vi "LOAD CELL MAIN CODE.vi"() -> ()   [LabVIEW 2025]
panel:
  in  "Case Constant\n(See Context Help) 3":bool=TRUE
  in  "Case Constant\n(See Context Help) 2":bool=TRUE
  in  "Case Constant\n(See Context Help)":bool
  in  "Acq Delay :":u32=20
  in  "FILE PATH":path
  in  "MODEL :":string
  out "LOAD CELL STATUS":bool
  in  "Start":bool=TRUE
  in  "stop":bool
  in  "Tab Control":T1(tab)
  in  "FILE NAME":string
  in  "Load cell parameter set":bool
  in  "SN":string="0"
  in  "ft_udp_handle":string="0"
  in  "PORT NO":string="8080"
  in  "IP ADDRESS":string="192.168.1.100"
  out "Fx":dbl(graph)
  out "Fy":dbl(graph)
  out "Fz":dbl(graph)
  out "Mx":dbl(graph)
  out "Mz":dbl(graph)
  out "My":dbl(graph)
  out "error out":errorcluster
  in  "error in (no error)":errorcluster
  out "model":string
  # "LOAD CELL DATA MONITOR"
types:
  T1 = enum32{"Instrument Details", "Fx", "Fy", "Fz", "Mx", "My", "Mz"}
  T2 = enum16{"INIT", "MAIN", "SET", "READ DATA", "CLOSE"}
  T3 = cluster{"load cell fgv ref":cluster{"Sensor IP":string, "Port":i32, "SN":i32, "model":string, "deleteHandle-result":i32, "initial-return":i32, "filter-return":i32, "zero-return":i32, "get-range-return":i32, "get-data-return":i32, "ft_udp_handle":i32, "ft_data":dbl[], "ft_range":dbl[], "running_flag":bool, "Create Handle":bool, "delete Handle":bool, "AE":bool, "uninitial-return":i32}, "main screen ref":cluster{"Fz":dbl, "Fy":dbl, "Fx":dbl, "Start":bool, "stop":bool, "IP ADDRESS":string, "PORT NO":string, "ft_udp_handle":string, "SN":string, "LOAD CELL STATUS":bool, "Load cell parameter set":bool, "FILE PATH":path, "MODEL :":string, "FILE NAME":string, "Tab Control":enum32{"Instrument Details", "Fx", "Fy", "Fz", "Mx", "My", "Mz"}, "Mz":dbl, "My":dbl, "Mx":dbl}}
  T4 = enum16{"INIT", "SETLOWPASSFILTER", "SETZERO", "GETSENSORINFO", "GETRANGE", "ZEROALL", "READDATA", "UNINITIAL", "DELETEHANDLE"}
  T5 = cluster{"Sensor IP":string, "Port":i32, "SN":i32, "model":string, "deleteHandle-result":i32, "initial-return":i32, "filter-return":i32, "zero-return":i32, "get-range-return":i32, "get-data-return":i32, "ft_udp_handle":i32, "ft_data":dbl[], "ft_range":dbl[], "running_flag":bool, "Create Handle":bool, "delete Handle":bool, "AE":bool, "uninitial-return":i32}
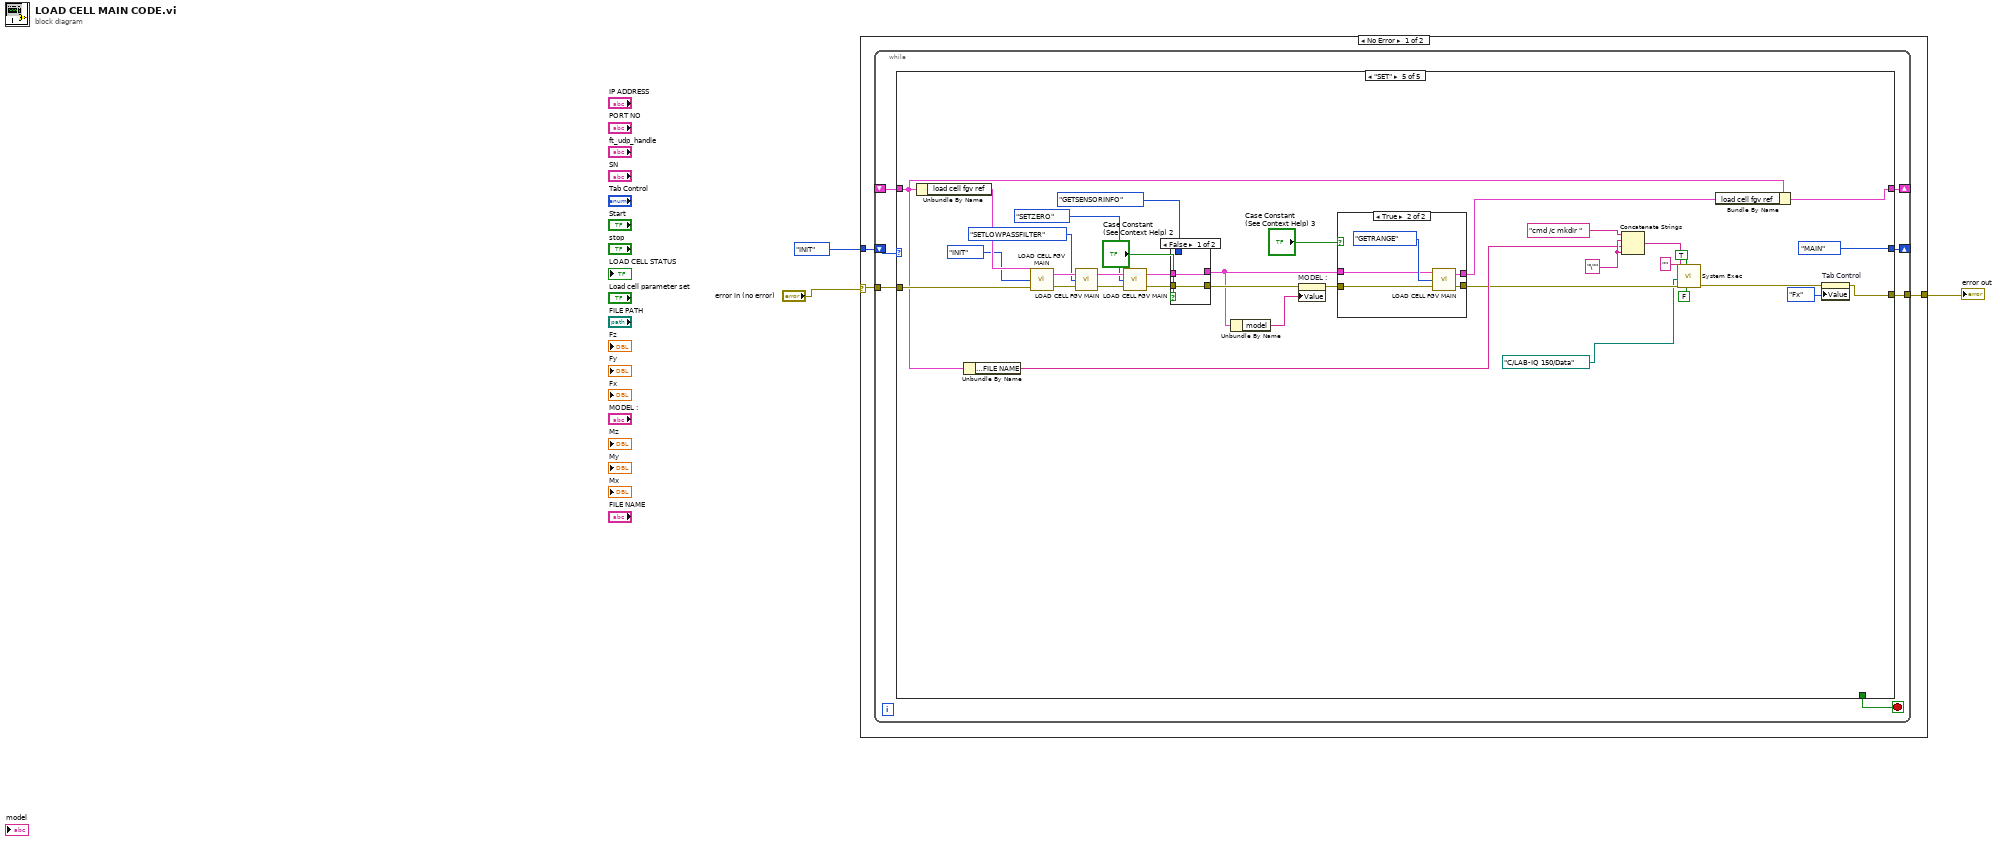
[diagram p0: block diagram]
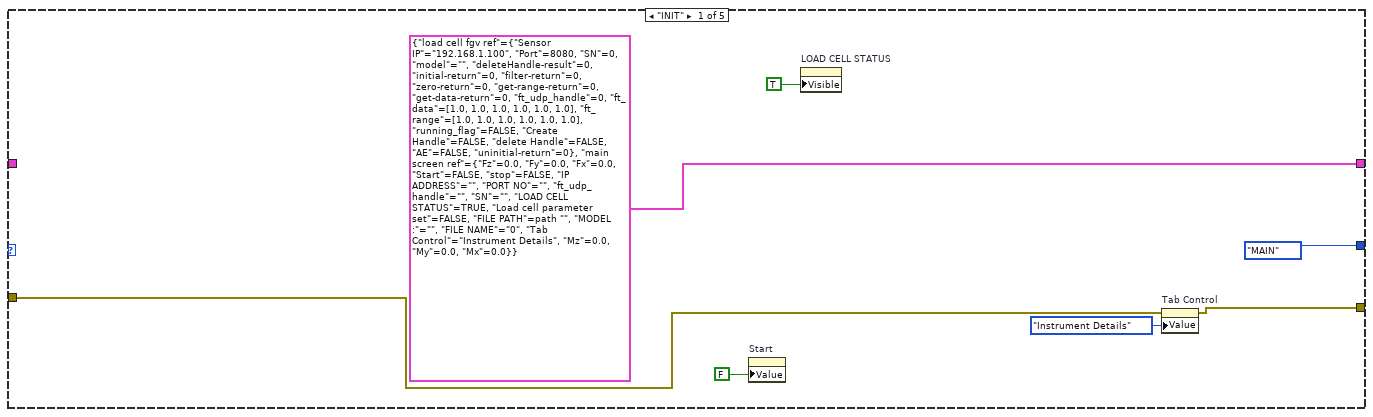
[diagram p2: hidden frame]
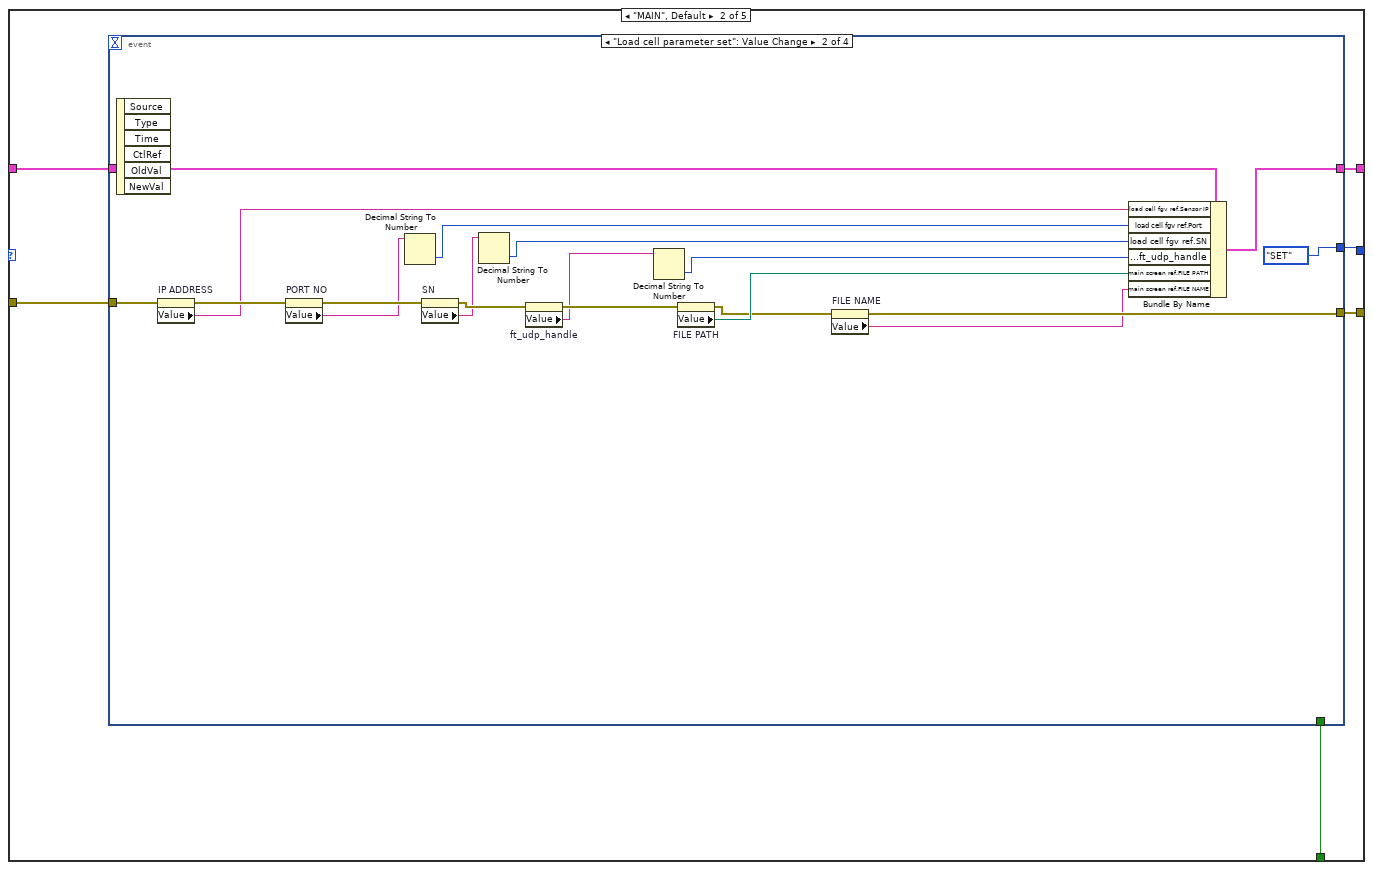
[diagram p3: hidden frame]
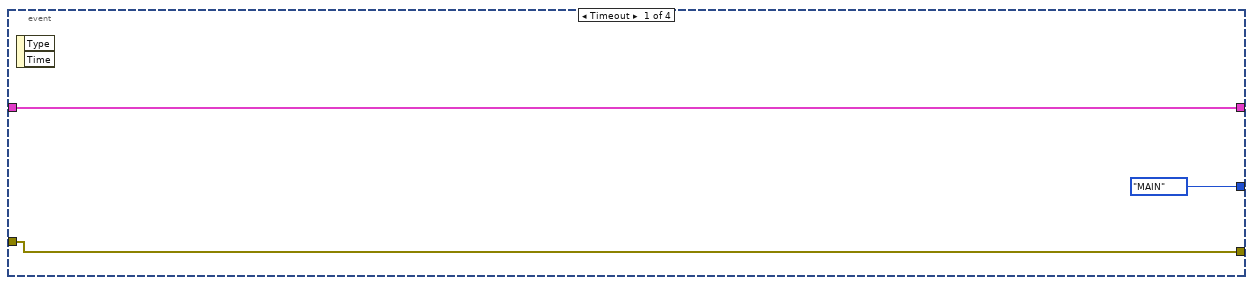
[diagram p4: hidden frame]
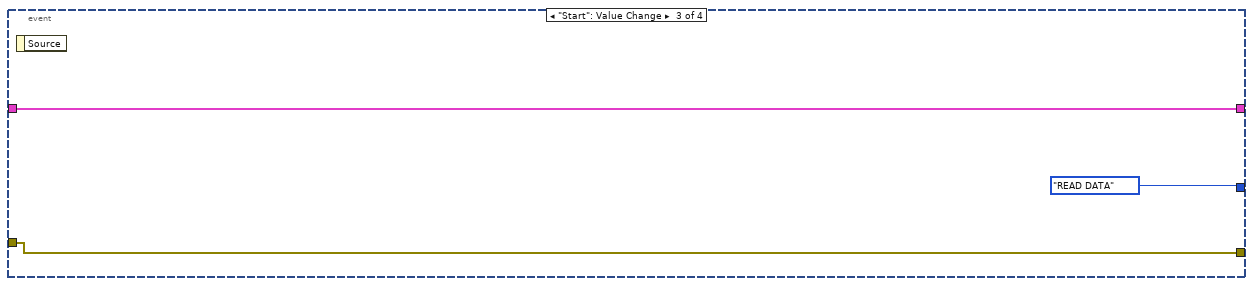
[diagram p5: hidden frame]
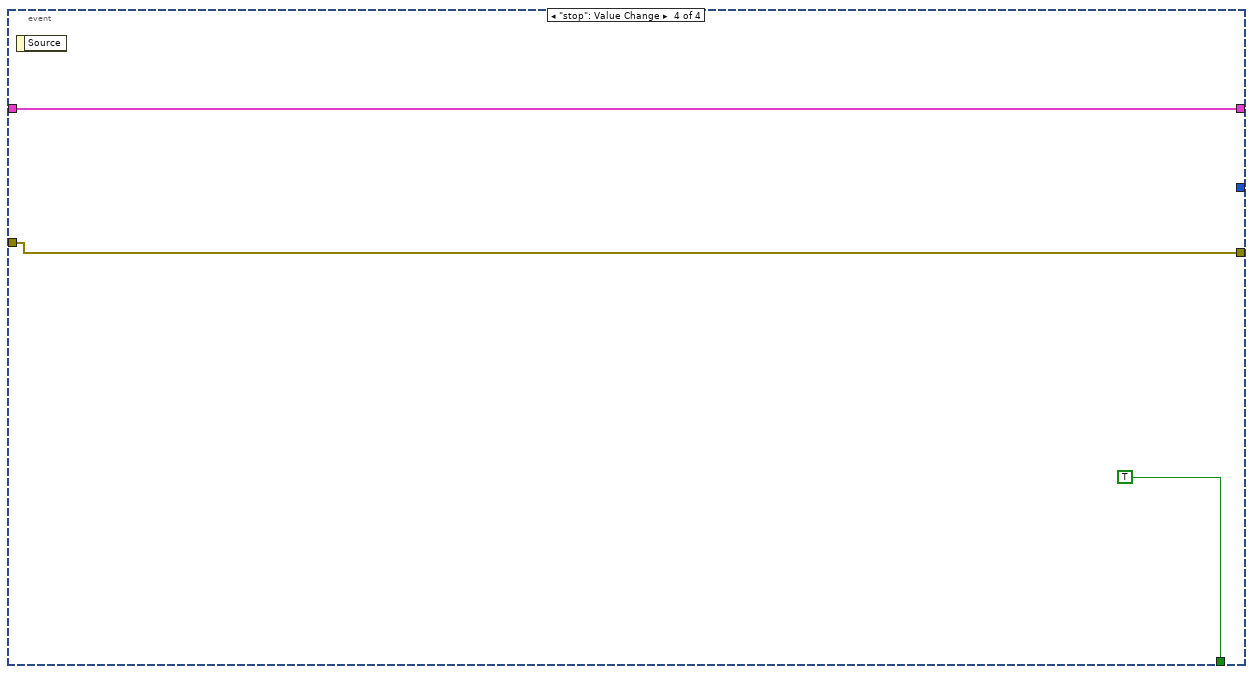
[diagram p6: hidden frame]
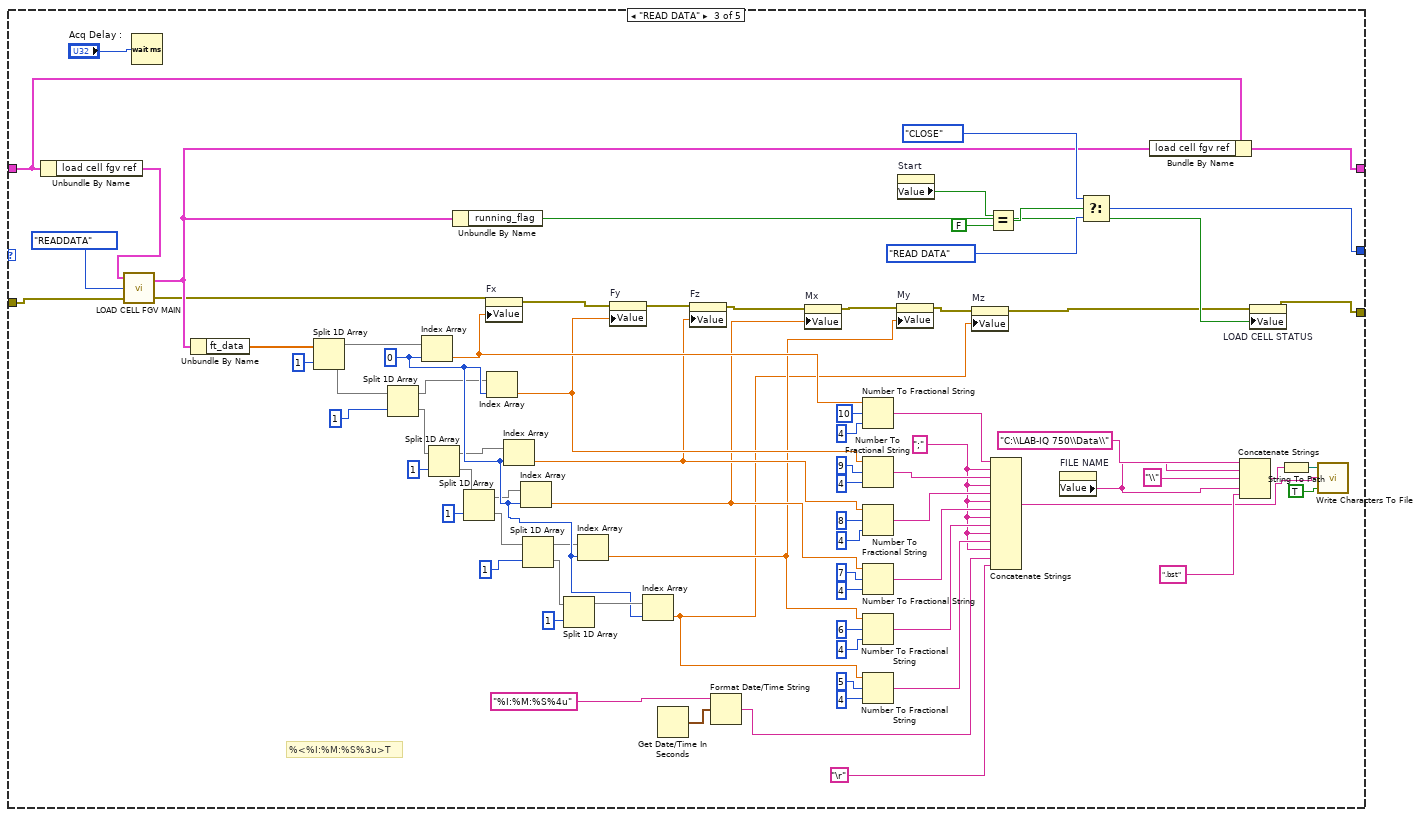
[diagram p7: hidden frame]
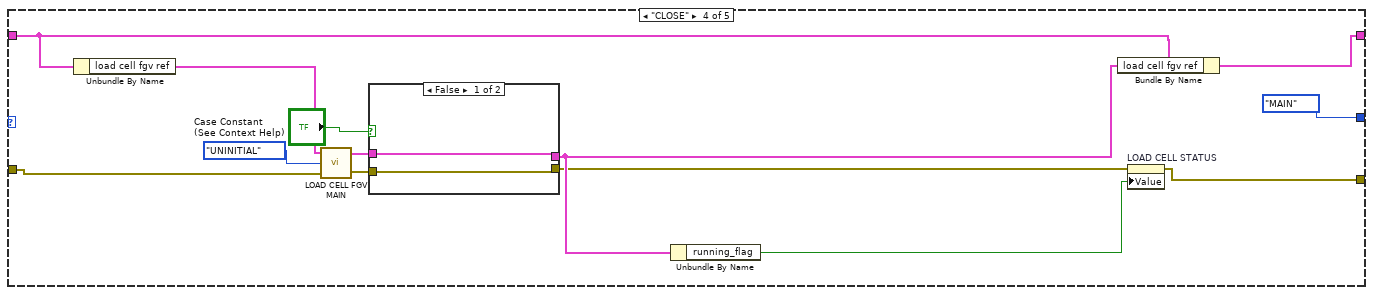
[diagram p8: hidden frame]
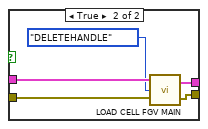
[diagram p9: hidden frame]
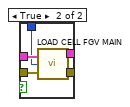
[diagram p11: hidden frame]
diagram:
  n1 = case shown="No Error" "error in (no error)" {
    selector: "error in (no error)" -> [w5 w201]
    tunnel: [w4 w201] -> w2
    tunnel: T2."INIT" -> [w6 _]
    frame No Error {
      n2 = while {
        shift-right: [w9] -> _
        shift-left: w6 -> [w13]
        tunnel: w5 -> [w12]
        shift-right: [w10] -> _
        shift-left: _ -> [w11]
        tunnel: [w8] -> w4
        stop <- w7 stop-if-true
        n3 = case shown="\"SET\"" w13 {
          tunnel: w12 -> [w17 w26 w132 w144 w186]
          tunnel: w11 -> [_ w23 w122 w142 w165]
          tunnel: [T3 {"load cell fgv ref"={"Sensor IP"="192.168.1.100", "Port"=8080, "SN"=0, "model"="", "deleteHandle-result"=0, "initial-return"=0, "filter-return"=0, "zero-return"=0, "get-range-return"=0, "get-data-return"=0, "ft_udp_handle"=0, "ft_data"=[1.0, 1.0, 1.0, 1.0, 1.0, 1.0], "ft_range"=[1.0, 1.0, 1.0, 1.0, 1.0, 1.0], "running_flag"=FALSE, "Create Handle"=FALSE, "delete Handle"=FALSE, "AE"=FALSE, "uninitial-return"=0}, "main screen ref"={"Fz"=0.0, "Fy"=0.0, "Fx"=0.0, "Start"=FALSE, "stop"=FALSE, "IP ADDRESS"="", "PORT NO"="", "ft_udp_handle"="", "SN"="", "LOAD CELL STATUS"=TRUE, "Load cell parameter set"=FALSE, "FILE PATH"=path "", "MODEL :"="", "FILE NAME"="0", "Tab Control"=enum."Instrument Details", "Mz"=0.0, "My"=0.0, "Mx"=0.0}} w24 w123 w141 w178] -> w10
          tunnel: [T2."MAIN" w25 w124 T2."MAIN" T2."MAIN"] -> w9
          tunnel: [w18 w22 w113 w134 w166] -> w8
          tunnel: [_ w21 _ _ _] -> w7
          frame "INIT" {
            n4 = property on="Start" class="Bool (strict)"("Value"=FALSE ("Start")) -> ()  [unwired: 2 in, 2 out]
            n5 = property on="LOAD CELL STATUS" class="Bool (strict)"("Visible"=TRUE) -> ()  [unwired: 2 in, 2 out]
            n6 = property on="Tab Control" class="TabCtl (strict)"(error in=w17, "Value"=enum32{"Instrument Details", "Fx", "Fy", "Fz"}."Instrument Details" ("Tab Control")) -> (error out=w18:errorcluster)  [unwired: 1 in, 1 out]
          }
          frame "MAIN", Default {
            n7 = event shown="[1] \"Load cell parameter set\": Value Change" {
              selector: _ -> [_ _ _ _]
              dyn-events: _ -> [_ _ _ _]
              timeout: _ -> [_ _ _ _]
              tunnel: w26 -> [w28 w48 w51 w54]
              tunnel: [T2."MAIN" T2."SET" T2."READ DATA" _] -> w25
              tunnel: [w27 w42 w49 w52] -> w24
              tunnel: w23 -> [w27 w43 w49 w52]
              tunnel: [w28 w37 w51 w54] -> w22
              tunnel: [_ _ _ TRUE] -> w21
              event Timeout {
                n8 = event-data() -> ()  [unwired: 1 in, 2 out]
              }
              event "Load cell parameter set": Value Change {
                n9 = event-data() -> ()  [unwired: 1 in, 6 out]
                n10 = property on="IP ADDRESS" class="Str"(error in=w48) -> (error out=w47:errorcluster, "Value"=w40:string)  [unwired: 1 in, 1 out]
                n11 = property on="PORT NO" class="Str"(error in=w47) -> (error out=w46:errorcluster, "Value"=w35:string)  [unwired: 1 in, 1 out]
                n12 = Decimal String To Number(string=w35) -> (number=w33:i32)  [unwired: 2 in, 1 out]
                n13 = property on="SN" class="Str"(error in=w46) -> (error out=w45:errorcluster, "Value"=w34:string)  [unwired: 1 in, 1 out]
                n14 = Decimal String To Number(string=w34) -> (number=w32:i32)  [unwired: 2 in, 1 out]
                n15 = property on="ft_udp_handle" class="Str"(error in=w45) -> (error out=w44:errorcluster, "Value"=w31:string)  [unwired: 1 in, 1 out]
                n16 = Decimal String To Number(string=w31) -> (number=w30:i32)  [unwired: 2 in, 1 out]
                n17 = property on="FILE PATH" class="Path"(error in=w44) -> (error out=w38:errorcluster, "Value"=w41:path)  [unwired: 1 in, 1 out]
                n18 = property on="FILE NAME" class="Str"(error in=w38) -> (error out=w37:errorcluster, "Value"=w36:string)  [unwired: 1 in, 1 out]
                n19 = Bundle By Name(cluster=w43, "load cell fgv ref.Sensor IP"=w40, "load cell fgv ref.Port"=w33, "load cell fgv ref.SN"=w32, "load cell fgv ref.ft_udp_handle"=w30, "main screen ref.FILE PATH"=w41, "main screen ref.FILE NAME"=w36) -> (w42:T3)
              }
              event "Start": Value Change {
                n20 = event-data() -> ()  [unwired: 1 in, 1 out]
              }
              event "stop": Value Change {
                n21 = event-data() -> ()  [unwired: 1 in, 1 out]
              }
            }
          }
          frame "READ DATA" {
            w59 = ";" ("F-format string")
            w71 = 0 ("index")
            # "%<%I:%M:%S%3u>T"
            n22 = Unbundle By Name(w122) -> ("load cell fgv ref"=w130:T5)
            n23 = call "LOAD CELL FGV MAIN.vi"("error in (no error)"=w132, "Enum"=T4."READDATA", "Cluster IN 2"=w130) -> ("error IO"=w110:errorcluster, "Cluster IN"=w114:T5)
            n24 = Wait (ms)(milliseconds to wait="Acq Delay :") -> ()  [unwired: 1 out]
            n25 = Unbundle By Name(w114) -> ("ft_data"=w117:dbl[])
            n26 = Split 1D Array(array=w117, index=1) -> (first subarray=w116:dbl[], second subarray=w121:dbl[])
            n27 = Split 1D Array(array=w121, index=1) -> (first subarray=w63:dbl[], second subarray=w115:dbl[])
            n28 = Index Array(array=w116, index=w71) -> (element=w89:dbl)
            n29 = Split 1D Array(array=w115, index=1) -> (first subarray=w62:dbl[], second subarray=w90:dbl[])
            n30 = Unbundle By Name(w114) -> ("running_flag"=w112:bool)
            n31 = Split 1D Array(array=w90, index=1) -> (first subarray=w61:dbl[], second subarray=w74:dbl[])
            n32 = property on="Fx" class="WFChart (strict)"(error in=w110, "Value"=w89) -> (error out=w109:errorcluster)  [unwired: 1 in, 1 out]
            n33 = Index Array(array=w63, index=w71) -> (element=w80:dbl)
            n34 = Index Array(array=w62, index=w71) -> (element=w79:dbl)
            n35 = Index Array(array=w61, index=w71) -> (element=w70:dbl)
            n36 = Split 1D Array(array=w74, index=1) -> (first subarray=w60:dbl[], second subarray=w73:dbl[])
            n37 = Split 1D Array(array=w73, index=1) -> (first subarray=w72:dbl[])  [unwired: 1 out]
            n38 = Index Array(array=w60, index=w71) -> (element=w69:dbl)
            n39 = property on="Fy" class="WFChart (strict)"(error in=w109, "Value"=w80) -> (error out=w108:errorcluster)  [unwired: 1 in, 1 out]
            n40 = Index Array(array=w72, index=w71) -> (element=w68:dbl)
            n41 = Get Date/Time In Seconds() -> (seconds since 1Jan1904=w57:timestamp)
            n42 = property on="Fz" class="WFChart (strict)"(error in=w108, "Value"=w79) -> (error out=w78:errorcluster)  [unwired: 1 in, 1 out]
            n43 = Format Date/Time String(time format string (%c)="%I:%M:%S%4u", seconds (now)=w57) -> (date/time string=w55:string)  [unwired: 1 in]
            n44 = property on="Mx" class="WFChart (strict)"(error in=w78, "Value"=w70) -> (error out=w77:errorcluster)  [unwired: 1 in, 1 out]
            n45 = Number To Fractional String(number=w89, width (-)=i16 10 ("precision (6)"), precision (6)=i16 4) -> (F-format string=w98:string)  [unwired: 1 in]
            n46 = Number To Fractional String(number=w80, width (-)=i16 9 ("precision (6)"), precision (6)=i16 4) -> (F-format string=w99:string)  [unwired: 1 in]
            n47 = Number To Fractional String(number=w79, width (-)=i16 8 ("precision (6)"), precision (6)=i16 4) -> (F-format string=w67:string)  [unwired: 1 in]
            n48 = Number To Fractional String(number=w70, width (-)=i16 7 ("precision (6)"), precision (6)=i16 4) -> (F-format string=w66:string)  [unwired: 1 in]
            n49 = Number To Fractional String(number=w69, width (-)=i16 6 ("precision (6)"), precision (6)=i16 4) -> (F-format string=w65:string)  [unwired: 1 in]
            n50 = Number To Fractional String(number=w68, width (-)=i16 5 ("precision (6)"), precision (6)=i16 4) -> (F-format string=w64:string)  [unwired: 1 in]
            n51 = property on="My" class="WFChart (strict)"(error in=w77, "Value"=w69) -> (error out=w76:errorcluster)  [unwired: 1 in, 1 out]
            n52 = property on="Start" class="Bool (strict)"() -> ("Value"=w129:bool)  [unwired: 2 in, 2 out]
            n53 = property on="Mz" class="WFChart (strict)"(error in=w76, "Value"=w68) -> (error out=w75:errorcluster)  [unwired: 1 in, 1 out]
            n54 = Equal?(x=w129, y=FALSE) -> (x = y?=w127:bool)
            n55 = Concatenate Strings(w98, w59, w99, w59, w67, w59, w66, w59, w65, w59, w64, w59, w55, "\r") -> (w94:string)
            n56 = property on="FILE NAME" class="Str"() -> ("Value"=w105:string)  [unwired: 2 in, 2 out]
            n57 = Select(t=T2."CLOSE", s=w127, f=T2."READ DATA") -> (s? t:f=w124:T2)
            n58 = Bundle By Name(cluster=w122, "load cell fgv ref"=w114) -> (w123:T3)
            n59 = Concatenate Strings("C:\\LAB-IQ 750\\Data\\" ("Substring"), w105, "\\" ("string"), w105, ".bst" ("Substring")) -> (w101:string)
            n60 = property on="LOAD CELL STATUS" class="Bool (strict)"(error in=w75, "Value"=w112) -> (error out=w113:errorcluster)  [unwired: 1 in, 1 out]
            n61 = String To Path(string=w101) -> (path=w102:path)
            n62 = call <vilib>:"Write Characters To File.vi"("append to file? (new file:F)"=TRUE, "character string"=w94, "file path (dialog if empty)"=w102) -> ()  [unwired: 2 in, 1 out]
          }
          frame "CLOSE" {
            n63 = Unbundle By Name(w142) -> ("load cell fgv ref"=w143:T5)
            n64 = call "LOAD CELL FGV MAIN.vi"("error in (no error)"=w144, "Enum"=T4."UNINITIAL", "Cluster IN 2"=w143) -> ("error IO"=w139:errorcluster, "Cluster IN"=w138:T5)
            n65 = case shown="False" "Case Constant\n(See Context Help)" {
              tunnel: w139 -> [w147 w152]
              tunnel: w138 -> [w146 w151]
              tunnel: [w146 w149] -> w137
              tunnel: [w147 w148] -> w136
              frame False {
              }
              frame True {
                n66 = call "LOAD CELL FGV MAIN.vi"("error in (no error)"=w152, "Enum"=T4."DELETEHANDLE", "Cluster IN 2"=w151) -> ("error IO"=w148:errorcluster, "Cluster IN"=w149:T5)
              }
            }
            n67 = Unbundle By Name(w137) -> ("running_flag"=w135:bool)
            n68 = Bundle By Name(cluster=w142, "load cell fgv ref"=w137) -> (w141:T3)
            n69 = property on="LOAD CELL STATUS" class="Bool (strict)"(error in=w136, "Value"=w135) -> (error out=w134:errorcluster)  [unwired: 1 in, 1 out]
          }
          frame "SET" {
            w164 = "\"" ("string")
            n70 = Unbundle By Name(w165) -> ("load cell fgv ref"=w185:T5)
            n71 = Unbundle By Name(w165) -> ("main screen ref.FILE NAME"=w158:string)
            n72 = call "LOAD CELL FGV MAIN.vi"("error in (no error)"=w186, "Enum"=T4."INIT", "Cluster IN 2"=w185) -> ("error IO"=w183:errorcluster, "Cluster IN"=w182:T5)
            n73 = call "LOAD CELL FGV MAIN.vi"("error in (no error)"=w183, "Enum"=T4."SETLOWPASSFILTER", "Cluster IN 2"=w182) -> ("error IO"=w174:errorcluster, "Cluster IN"=w181:T5)
            n74 = call "LOAD CELL FGV MAIN.vi"("error in (no error)"=w174, "Enum"=T4."SETZERO", "Cluster IN 2"=w181) -> ("error IO"=w173:errorcluster, "Cluster IN"=w180:T5)
            n75 = case shown="False" "Case Constant\n(See Context Help) 2" {
              tunnel: w180 -> [w194 w200]
              tunnel: T4."GETSENSORINFO" ("Enum") -> [_ w199]
              tunnel: w173 -> [w195 w198]
              tunnel: [w195 w197] -> w172
              tunnel: [w194 w196] -> w170
              frame False {
              }
              frame True {
                n76 = call "LOAD CELL FGV MAIN.vi"("error in (no error)"=w198, "Enum"=w199, "Cluster IN 2"=w200) -> ("error IO"=w197:errorcluster, "Cluster IN"=w196:T5)
              }
            }
            n77 = Unbundle By Name(w170) -> ("model"=w169:string)
            n78 = property on="MODEL :" class="Str"(error in=w172, "Value"=w169) -> (error out=w171:errorcluster)  [unwired: 1 in, 1 out]
            n79 = case shown="True" "Case Constant\n(See Context Help) 3" {
              tunnel: [w187 w193] -> w179
              tunnel: w171 -> [w188 w191]
              tunnel: w170 -> [w187 w190]
              tunnel: [w188 w189] -> w157
              frame False {
              }
              frame True {
                n80 = call "LOAD CELL FGV MAIN.vi"("error in (no error)"=w191, "Enum"=T4."GETRANGE", "Cluster IN 2"=w190) -> ("error IO"=w189:errorcluster, "Cluster IN"=w193:T5)
              }
            }
            n81 = Concatenate Strings("cmd /c mkdir " ("string"), w164, w158, w164) -> (w160:string)
            n82 = call <vilib>:"System Exec.vi"("run minimized? (F)"=FALSE, "wait until completion? (T)"=TRUE, "error in (no error)"=w157, "working directory"=path "C:/LAB-IQ 150/Data", "standard input"="", "command line"=w160) -> ("error out"=w156:errorcluster)  [unwired: 2 in, 3 out]
            n83 = Bundle By Name(cluster=w165, "load cell fgv ref"=w179) -> (w178:T3)
            n84 = property on="Tab Control" class="TabCtl (strict)"(error in=w156, "Value"=enum32{"Instrument Details", "Fx", "Fy", "Fz"}."Fx" ("Tab Control")) -> (error out=w166:errorcluster)  [unwired: 1 in, 1 out]
          }
        }
      }
    }
    frame Error {
    }
  }
  "error out" <- w2
